vi "ProcessInputs.vi"(8 "error in (no error)":errorcluster, 10 "Destination Directory":path, 11 "Source directory/files":path) -> (0 "error out":errorcluster, 1 "Continue?":bool, 2 "Destination Directory out":path, 3 "Source directory/files out":path)   [LabVIEW 2017]
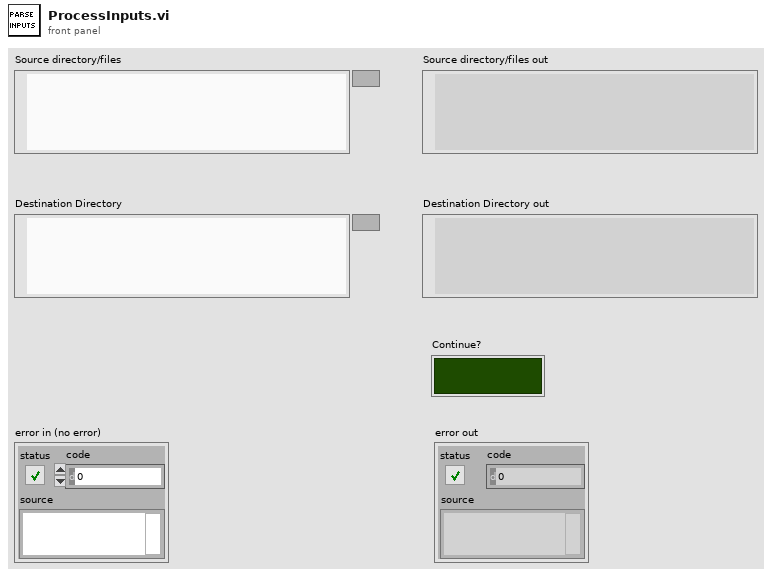
[diagram p1: front panel]
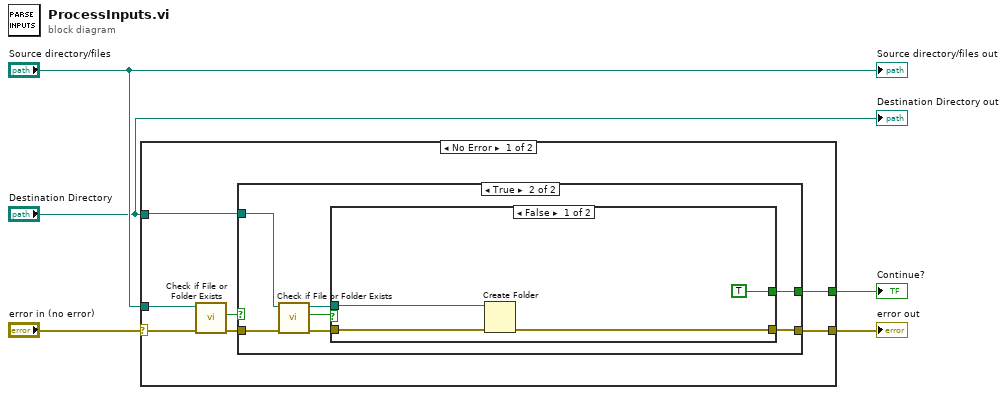
[diagram p0: block diagram]
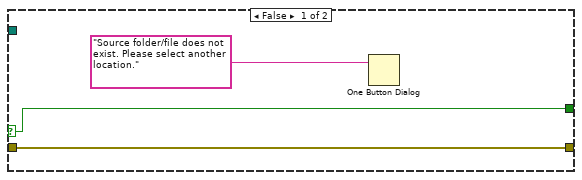
[diagram p2: hidden frame]
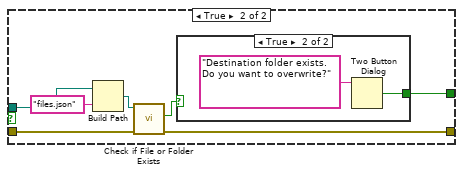
[diagram p3: hidden frame]
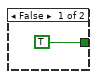
[diagram p4: hidden frame]
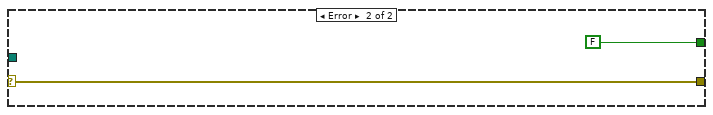
[diagram p5: hidden frame]
diagram:
  n1 = case shown="No Error" "error in (no error)" {
    selector: "error in (no error)" -> [w12 w37]
    tunnel: [w9 FALSE] -> w4
    tunnel: "Source directory/files" -> [w10 _]
    tunnel: "Destination Directory" -> [w8 _]
    tunnel: [w11 w37] -> w1
    frame No Error {
      n2 = call <vilib>:"Check if File or Folder Exists.vi"("error in (no error)"=w12, "path"=w10) -> ("error out"=w6:errorcluster, "file or folder exists?"=w7:bool)  [unwired: 7 in, 1 out]
      n3 = case shown="True" w7 {
        selector: w7 -> [w15 _]
        tunnel: [w15 w19] -> w9
        tunnel: w6 -> [w13 w21]
        tunnel: w8 -> [_ w20]
        tunnel: [w13 w16] -> w11
        frame False {
          n4 = One Button Dialog(message="Source folder/file does not exist. Please select another location.") -> ()  [unwired: 1 in, 1 out]
        }
        frame True {
          n5 = call <vilib>:"Check if File or Folder Exists.vi"("error in (no error)"=w21, "path"=w20) -> ("error out"=w17:errorcluster, "file or folder exists?"=w22:bool, "dup path"=w18:path)  [unwired: 7 in]
          n6 = case shown="False" w22 {
            tunnel: [TRUE ("T button?") w33] -> w19
            tunnel: w18 -> [w25 w32]
            tunnel: w17 -> [w24 w28]
            tunnel: [w23 w27] -> w16
            frame False {
              n7 = Create Folder(path (use dialog)=w25, error in=w24) -> (error out=w23:errorcluster)  [unwired: 1 in, 2 out]
            }
            frame True {
              n8 = Build Path(base path=w32, name or relative path="files.json") -> (appended path=w30:path)
              n9 = call <vilib>:"Check if File or Folder Exists.vi"("error in (no error)"=w28, "path"=w30) -> ("error out"=w27:errorcluster, "file or folder exists?"=w29:bool)  [unwired: 7 in, 1 out]
              n10 = case shown="True" w29 {
                tunnel: [TRUE ("T button?") w35] -> w33
                frame False {
                }
                frame True {
                  n11 = Two Button Dialog(message="Destination folder exists. Do you want to overwrite?") -> (T button?=w35:bool)  [unwired: 2 in]
                }
              }
            }
          }
        }
      }
    }
    frame Error {
    }
  }
  "Continue?" <- w4
  "error out" <- w1
  "Source directory/files out" <- "Source directory/files"
  "Destination Directory out" <- "Destination Directory"
